vi "z-axis-manual.vi"() -> ()   [LabVIEW 2015]
uses:
  <vilib>/rvi/Emulation/niFpgaGetClockAttributes.vi
  <vilib>/rvi/Emulation/niFpgaSctlEmulationGetInTimedLoop.vi
  <vilib>/rvi/Emulation/niFpgaEmulationReportErrorSimple.vi
  <vilib>/rvi/eio/common/nirviEmuTemplateMethod_errors.vi
  <vilib>/rvi/Emulation/niFpgaCriticalErrorInLSC.vi
  <vilib>/eio/EIONode/EIONode.xnode
panel:
  in  "Mod1/AO2":fxp<+/-,20,5>
  in  "Boolean":bool=TRUE
  out "x-y":sgl
  in  "Cluster":cluster{"TsTicks":u32, "force setpoint":sgl}
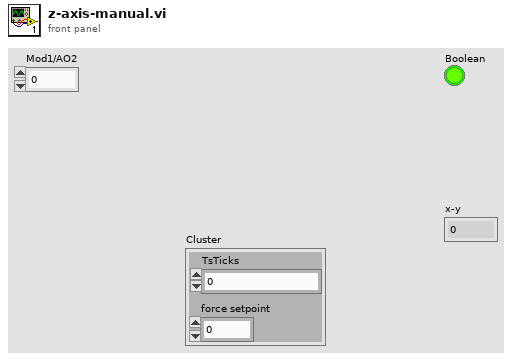
[diagram p1: front panel]
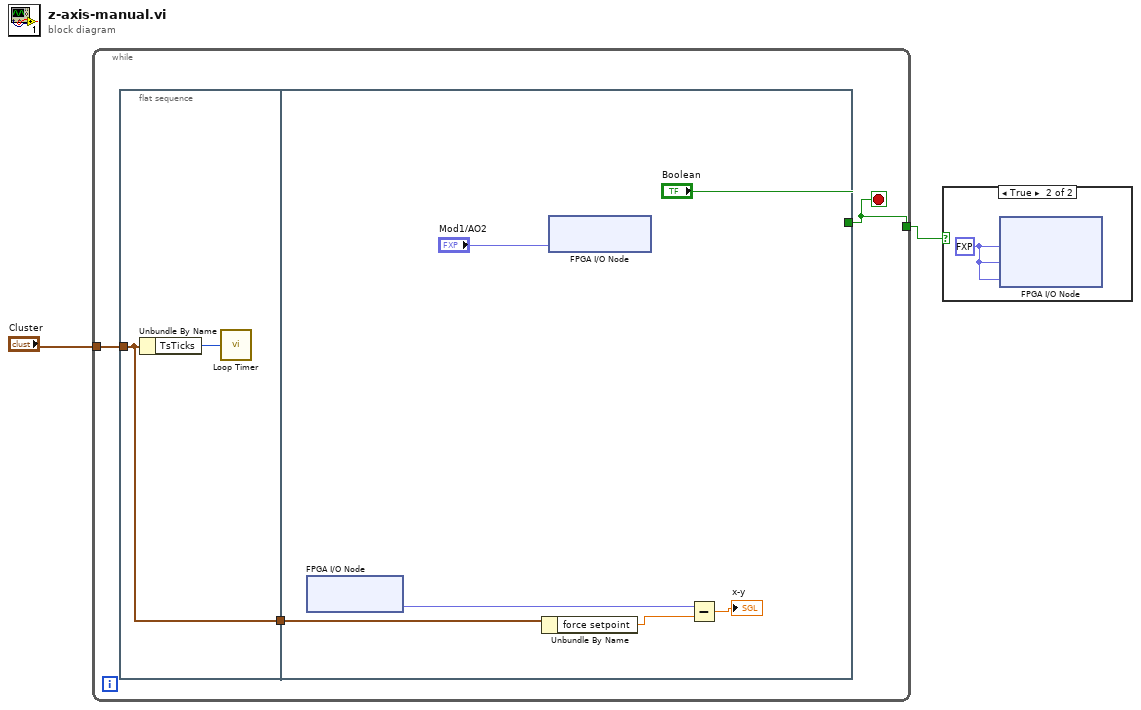
[diagram p0: block diagram]
diagram:
  n1 = while {
    tunnel: [w5] -> w1
    tunnel: "Cluster" -> [w4]
    stop <- w5 stop-if-true
    n2 = flat-sequence {
      tunnel: w4 -> [w6]
      tunnel: [w6] -> w3
      tunnel: ["Boolean"] -> w5
      tunnel: w3 -> [w13]
      frame #0 {
        n3 = Unbundle By Name(w6) -> ("TsTicks"=w7:u32)
        n4 = call "Loop Timer"("Count(Ticks)"=w7) -> ()  [unwired: 1 out]
      }
      frame #1 {
        n5 = xnode "FPGA I/O Node"() -> ("Mod2/AI2"=w9:fxp<+/-,24,5>)  [unwired: 1 in, 1 out]
        n6 = Unbundle By Name(w13) -> ("force setpoint"=w12:sgl)
        n7 = xnode "FPGA I/O Node"("Mod1/AO2"="Mod1/AO2") -> ()  [unwired: 1 in, 1 out]
        n8 = Subtract(x=w9, y=w12) -> (x-y=→"x-y":sgl)
      }
    }
  }
  n9 = case shown="True" w1 {
    frame False {
    }
    frame True {
      w14 = fxp<+/-,20,5> 0.0 ("Mod1/AO0")
      n10 = xnode "FPGA I/O Node"("Mod1/AO0"=w14, "Mod1/AO1"=w14, "Mod1/AO2"=w14) -> ()  [unwired: 3 in, 3 out]
    }
  }
